vi "Event case-Speed graph behaviour switch.vi"(8 "error in (no error)":errorcluster, 11 "Speed graph behaviour":T1) -> (0 "error out":errorcluster)   [LabVIEW 2017]
uses:
  Typedefs/Speed graph behaviour enum.ctl
  Functional Imaging Viewer/Typedefs/Get-Set-Clear Control.ctl
  Globals/gl_Time series viewer globals.vi
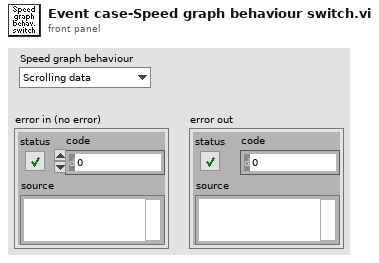
[diagram p1: front panel]
types:
  T1 = typedef "Speed graph behaviour enum.ctl" = enum16{"Scrolling data", "Scrolling cursor"}
  T2 = typedef "Get-Set-Clear Control.ctl" = enum16{"Get", "Set", "Clear"}
  T3 = typedef "Time series viewer refs.ctl" = cluster{"This VI":refnum<vi>, "Image control":refnum<vi>, "AVI Mode ind":refnum<vi>, "Play":refnum<vi>, "Stop":refnum<vi>, "Back":refnum<vi>, "Scrollbar":refnum<vi>, "Video length info":refnum<vi>, "Expected speed values":refnum<vi>, "Intensity":refnum<vi>, "Path":refnum<vi>, "Selection sliders":refnum<vi>, "Speed Graph ref":refnum<vi>, "Frame rate set (fps)":refnum<vi>, "Channel to load":refnum<vi>, "Number of rows to generate":refnum<vi>, "Colour":refnum<vi>}
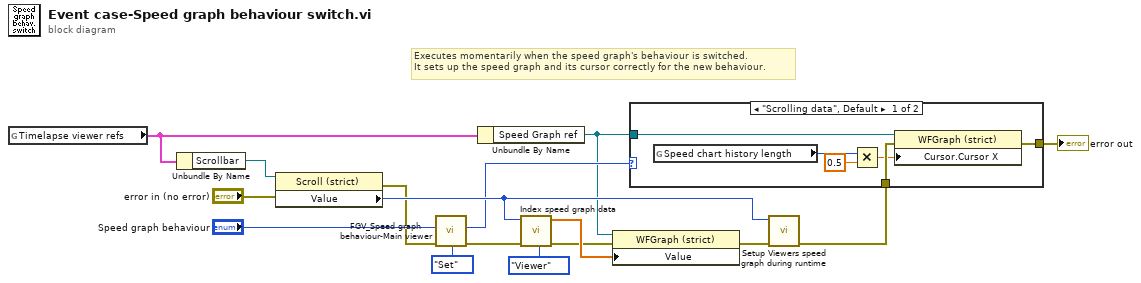
[diagram p0: block diagram]
diagram:
  # "Executes momentarily when the speed graph's behaviour is switched.\nIt sets up the speed graph and its cursor correctly for the new behaviour."
  n1 = global read "gl_Time series viewer globals.vi" "Timelapse viewer refs"() -> (w8:T3)
  n2 = Unbundle By Name(w8) -> ("Scrollbar"=w12:refnum<vi>)
  n3 = property class="Scroll (strict)"(reference=w12, error in="error in (no error)") -> (error out=w10:errorcluster, "Value"=w11:i32)  [unwired: 1 out]
  n4 = call "FGV_Speed graph behaviour-Main viewer.vi"("Function"=Get-Set-Clear_Control."Set", "error in (no error)"=w10, "Speed graph behaviour"="Speed graph behaviour") -> ("error out"=w13:errorcluster, "Speed graph behaviour"=w4:T1)  [unwired: 7 in]
  n5 = Unbundle By Name(w8) -> ("Speed Graph ref"=w1:refnum<vi>)
  n6 = call "Index speed graph data.vi"("Caller"=enum16{"Viewer", "Exporter"}."Viewer", "error in (no error)"=w13, "Gobal frame number in Timelapse data/master video (1 based)"=w11) -> ("error out"=w6:errorcluster, "Speed data waveform graph"=w7:dbl[])  [unwired: 6 in, 1 out]
  n7 = property class="WFGraph (strict)"(reference=w1, error in=w6, "Value"=w7) -> (error out=w5:errorcluster)  [unwired: 1 out]
  n8 = call "Setup Viewers speed graph during runtime.vi"("error in (no error)"=w5, "Frame number or cycle number"=w11) -> ("error out"=w3:errorcluster)  [unwired: 9 in]
  n9 = case shown="\"Scrolling data\", Default" w4 {
    tunnel: w3 -> [w20 w23]
    tunnel: [w19 w23] -> w2
    tunnel: w1 -> [w17 _]
    frame "Scrolling data", Default {
      n10 = global read "gl_Time series viewer globals.vi" "Speed chart history length"() -> (w21:i32)
      n11 = Multiply(x=w21, y=0.5) -> (x*y=w18:dbl)
      n12 = property on="Property Node" class="WFGraph (strict)"(reference=w17, error in=w20, "Cursor.Cursor X"=w18) -> (error out=w19:errorcluster)  [unwired: 1 out]
    }
    frame "Scrolling cursor" {
    }
  }
  "error out" <- w2
